vi "Set Analyze Parameter.vi"(8 "error in (no error)":errorcluster, 10 "Analyze Parameter":refnum<class "Analyze Parameter Base.lvclass">, 11 "Analyze Actor in":refnum<class "Analyze Actor.lvclass">) -> (0 "error out":errorcluster, 3 "Analyze Actor out":refnum<class "Analyze Actor.lvclass">)   [LabVIEW 2014, in "Analyze Actor.lvlib" / "Analyze Actor.lvclass"]
uses:
  Analyze Actor.lvclass
  Analyze Parameter/Analyze Parameter Base/Analyze Parameter Base.lvclass
  Analyze Actor.lvclass/Analyze Actor.ctl
  Analyze Classes/Analyze BaseClass/Analyze BaseClass/Analyze BaseClass.lvclass
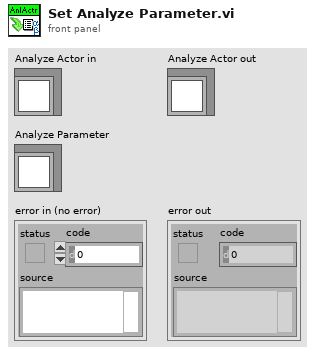
[diagram p1: front panel]
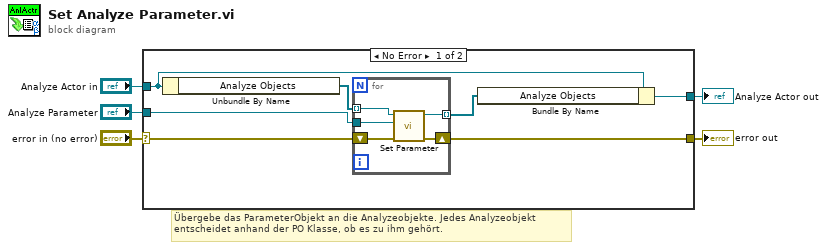
[diagram p0: block diagram]
diagram:
  # "Übergebe das ParameterObjekt an die Analyzeobjekte. Jedes Analyzeobjekt \nentscheidet anhand der PO Klasse, ob es zu ihm gehört."
  n1 = case shown="No Error" "error in (no error)" {
    selector: "error in (no error)" -> [w8 w19]
    tunnel: [w6 w19] -> w4
    tunnel: [w7 w18] -> w2
    tunnel: "Analyze Actor in" -> [w12 w18]
    tunnel: "Analyze Parameter" -> [w10 _]
    frame No Error {
      n2 = Unbundle By Name(w12) -> ("Analyze Objects"=w11:refnum<class "Analyze BaseClass.lvclass">[])
      n3 = for {
        tunnel: w11 -> [w17] mode=indexing
        tunnel: w10 -> [w16]
        tunnel: [w15] -> w9 mode=indexing
        shift-right: [w14] -> w6
        shift-left: w8 -> [w13]
        n4 = call "Set Parameter.vi"("error in (no error)"=w13, "Analyze Parameter"=w16, "Analyze BaseClass in"=w17) -> ("error out"=w14:errorcluster, "Analyze BaseClass out"=w15:refnum<class "Analyze BaseClass.lvclass">)  [unwired: 7 in]
      }
      n5 = Bundle By Name(cluster=w12, "Analyze Objects"=w9) -> (w7:refnum<class "Analyze Actor.lvclass">)
    }
    frame Error {
    }
  }
  "error out" <- w4
  "Analyze Actor out" <- w2
